vi "CAN_Init.vi"(8 "error in (no error)":errorcluster caption="错误输入（无错误）", 10 "VCI_INIT_CONFIG":T3={"AccCode"=0, "AccMask"=4294967295, "Reserved"=0, "Filter"=1, "Timing0"=9, "Timing1"=28, "Mode"=0} {"Timing1" format="%x"; "Timing0" format="%x"; "Filter" format="%x"; "AccMask" format="%x"}, 11 "General_Input":T2) -> (0 "错误输出":errorcluster, 3 "General_Output":T1)   [LabVIEW 2012]
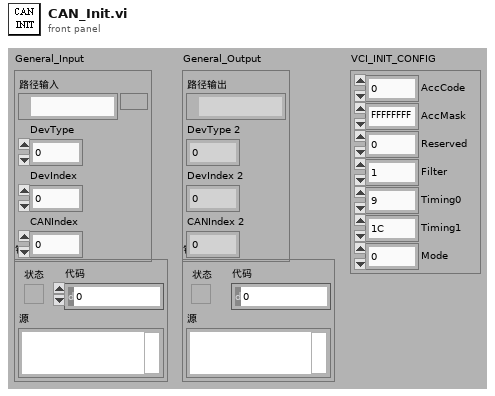
[diagram p1: front panel]
types:
  T1 = cluster{"路径输出":path, "DevType 2":u32, "DevIndex 2":u32, "CANIndex 2":u32}
  T2 = cluster{"路径输入":path, "DevType":u32, "DevIndex":u32, "CANIndex":u32}
  T3 = cluster{"AccCode":u32, "AccMask":u32, "Reserved":u32, "Filter":u8, "Timing0":u8, "Timing1":u8, "Mode":u8}
  T4 = cluster{"path out":path, "DevType":u32, "DevIndex":u32, "CANIndex":u32}
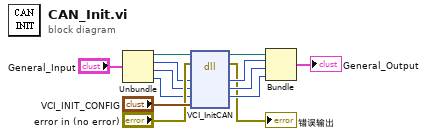
[diagram p0: block diagram]
diagram:
  n1 = Unbundle("General_Input") -> ("路径输入"=w10:path, "DevType"=w8:u32, "DevIndex"=w7:u32, "CANIndex"=w9:u32)
  n2 = dll-call lib="?" fn="VCI_InitCAN"(path in=w10, error in="error in (no error)", "DevType"=w8, "DevIndex"=w7, "CANIndex"=w9, "pInitConfig"="VCI_INIT_CONFIG") -> (path out=w6:path, error out=→"错误输出":errorcluster, "DevType"=w5:u32, "DevIndex"=w3:u32, "CANIndex"=w4:u32)  [unwired: 3 in]
  n3 = Bundle("path out"=w6, "DevType"=w5, "DevIndex"=w3, "CANIndex"=w4) -> (→"General_Output":T4)  [unwired: 1 in]
